vi "TEST Object Manual Bounds (By Reference Splitter).vi"() -> ()   [LabVIEW 2013, in "IObject.lvclass"]
uses:
  IObject.lvclass
  IContainer/Viewport/Viewport.lvclass
  IContainer/Divider/Splitter/Splitter.lvclass
  Interaction By Refererence/Interaction By Refererence.lvclass
  Object/Object.lvclass
panel:
  out "XY Graph 6":cluster{"X":dbl, "Y":dbl}[](graph)
  out "XY Graph 5":cluster{"X":dbl, "Y":dbl}[](graph)
  out "XY Graph 4":cluster{"X":dbl, "Y":dbl}[](graph)
  out "XY Graph 3":cluster{"X":dbl, "Y":dbl}[](graph)
  out "XY Graph 2":cluster{"X":dbl, "Y":dbl}[](graph)
  out "XY Graph":cluster{"X":dbl, "Y":dbl}[](graph)
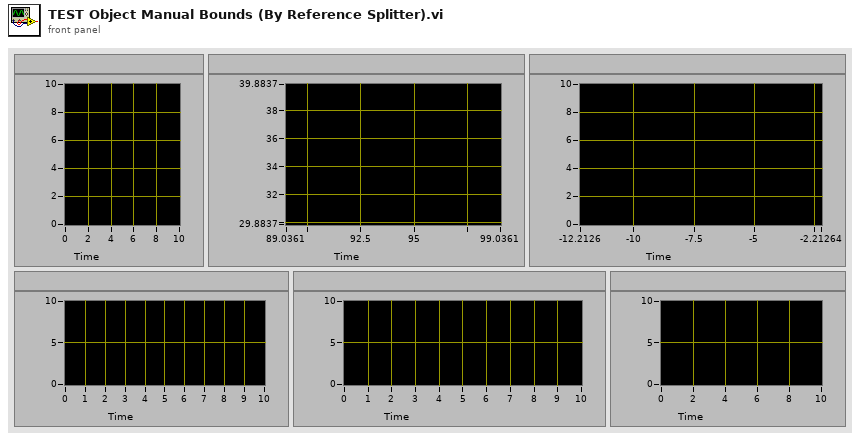
[diagram p1: front panel]
types:
  T1 = cluster{"Left":dbl, "Top":dbl, "Right":dbl, "Bottom":dbl}
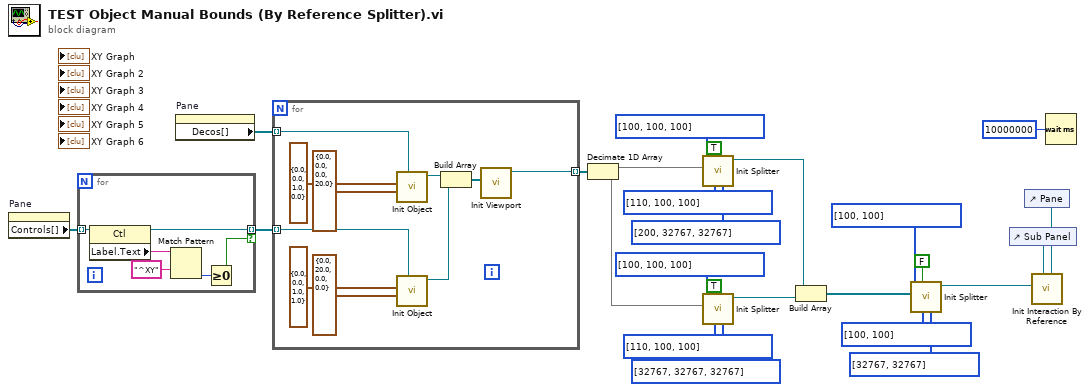
[diagram p0: block diagram]
diagram:
  n1 = property on="Pane" class="Pane"() -> ("Controls[]"=w5:refnum<vi>[])  [unwired: 2 in, 2 out]
  n2 = for {
    tunnel: w5 -> [w31] mode=indexing
    tunnel: [w28] -> w4 mode=indexing if=w26
    n3 = property class="Ctl"(reference=w31) -> (reference out=w28:refnum<vi>, "Label.Text"=w30:string)  [unwired: 1 in, 1 out]
    n4 = Match Pattern(string=w30, regular expression="^XY") -> (offset past match=w27:i32)  [unwired: 1 in, 3 out]
    n5 = Greater Or Equal To 0?(x=w27) -> (x >= 0?=w26:bool)
  }
  n6 = property on="Pane" class="Pane"() -> ("Decos[]"=w24:refnum<vi>[])  [unwired: 2 in, 2 out]
  n7 = for {
    tunnel: w24 -> [w41] mode=indexing
    tunnel: [w32] -> w18 mode=indexing
    tunnel: w4 -> [w35] mode=indexing
    n8 = call "Init Object.vi"("GObj Refnum"=w41, "B [0, 0, 0, 0]"=T1 {"Left"=0.0, "Top"=0.0, "Right"=0.0, "Bottom"=20.0} ("B"), "A [0, 0, 1, 1]"=T1 {"Left"=0.0, "Top"=0.0, "Right"=1.0, "Bottom"=0.0} ("A")) -> ("MMI Scaling out"=w34:refnum<class "Object.lvclass">)  [unwired: 7 in, 1 out]
    n9 = call "Init Object.vi"("GObj Refnum"=w35, "B [0, 0, 0, 0]"=T1 {"Left"=0.0, "Top"=20.0, "Right"=0.0, "Bottom"=0.0} ("B"), "A [0, 0, 1, 1]"=T1 {"Left"=0.0, "Top"=0.0, "Right"=1.0, "Bottom"=1.0} ("A")) -> ("MMI Scaling out"=w33:refnum<class "Object.lvclass">)  [unwired: 7 in, 1 out]
    n10 = Build Array(w34, w33) -> (w38:refnum<class "Object.lvclass">[])
    n11 = call "Init Viewport.vi"("Items"=w38) -> ("Viewport out"=w32:refnum<class "Viewport.lvclass">)  [unwired: 9 in, 1 out]
  }
  n12 = Decimate 1D Array(w18) -> (w19:refnum<class "Viewport.lvclass">[], w12:refnum<class "Viewport.lvclass">[])
  n13 = call "Init Splitter.vi"("Maximal size"=i16[] [200, 32767, 32767] ("Minimal size"), "Minimal size"=i16[] [110, 100, 100], "Vertical? [F, hor.]"=TRUE, "Relative size"=i16[] [100, 100, 100] ("Minimal size"), "Items"=w19) -> ("Splitter out"=w25:refnum<class "Splitter.lvclass">)  [unwired: 5 in, 1 out]
  n14 = call "Init Splitter.vi"("Maximal size"=i16[] [32767, 32767, 32767] ("Minimal size"), "Minimal size"=i16[] [110, 100, 100], "Vertical? [F, hor.]"=TRUE, "Relative size"=i16[] [100, 100, 100] ("Minimal size"), "Items"=w12) -> ("Splitter out"=w13:refnum<class "Splitter.lvclass">)  [unwired: 5 in, 1 out]
  n15 = Build Array(w25, w13) -> (w11:refnum<class "Splitter.lvclass">[])
  n16 = call "Init Splitter.vi"("Maximal size"=i16[] [32767, 32767] ("Size"), "Minimal size"=i16[] [100, 100] ("Size"), "Vertical? [F, hor.]"=FALSE, "Relative size"=i16[] [100, 100] ("Size"), "Items"=w11) -> ("Splitter out"=w6:refnum<class "Splitter.lvclass">)  [unwired: 5 in, 1 out]
  n17 = control-ref of="Sub Panel"() -> (w3:refnum<vi>)
  n18 = control-ref of="Pane"() -> (w2:refnum<vi>)
  n19 = call "Init Interaction By Reference.vi"("Pane"=w2, "Sub Panel"=w3, "IObject"=w6) -> ()  [unwired: 6 in, 3 out]
  n20 = Wait (ms)(milliseconds to wait=u32 10000000) -> ()  [unwired: 1 out]
